vi "Peak.vi"(8 "error in (no error)":errorcluster, 11 "TypedCircularBuffer in":refnum<class "RotateCircularBuffer.lvclass">) -> (0 "error out":errorcluster, 2 "element":T1, 3 "TypedCircularBuffer out":refnum<class "RotateCircularBuffer.lvclass">)   [LabVIEW 2024, in "RotateCircularBuffer.lvclass"]
uses:
  RotateCircularBuffer.lvclass
  Type.ctl
  RotateCircularBuffer.lvclass/RotateCircularBuffer.ctl
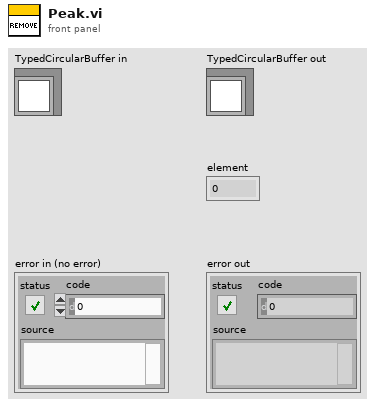
[diagram p1: front panel]
types:
  T1 = typedef "RotateCircularBuffer.lvclass/Type.ctl" = u8
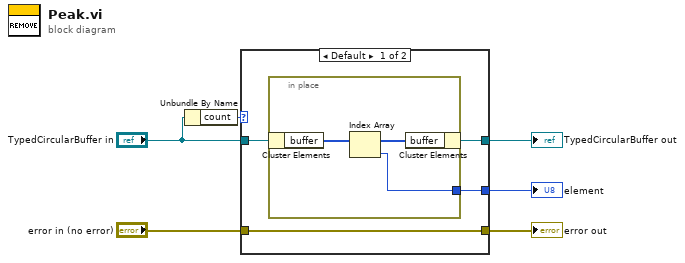
[diagram p0: block diagram]
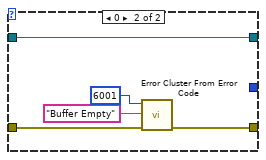
[diagram p2: hidden frame]
diagram:
  n1 = Unbundle By Name("TypedCircularBuffer in") -> ("count"=w1:u32)
  n2 = case shown="Default" w1 {
    tunnel: "error in (no error)" -> [w9 w17]
    tunnel: [w9 w16] -> w5
    tunnel: "TypedCircularBuffer in" -> [w10 w13]
    tunnel: [w8 w13] -> w3
    tunnel: [w7 _] -> w2
    frame Default {
      n3 = in-place {
        in-place-border: [w11] -> w7
        n4 = in-place-cluster #1(w10) -> ("buffer"=w12:T1[])
        n5 = Index Array(array=w12) -> (element=w11:T1)  [unwired: 1 in]
        n6 = in-place-cluster #1("buffer"=w12) -> (w8:refnum<class "RotateCircularBuffer.lvclass">)
      }
    }
    frame 0 {
      n7 = call <vilib>:"Error Cluster From Error Code.vi"("error in (no error)"=w17, "error message (\"\")"="Buffer Empty" ("error message (\"\")"), "error code (0)"=6001) -> ("error out"=w16:errorcluster)  [unwired: 6 in]
    }
  }
  "TypedCircularBuffer out" <- w3
  "error out" <- w5
  "element" <- w2
